vi "LabVIEW-Demo.vi"() -> ()   [LabVIEW 2015]
uses:
  <vilib>/Math Plots/3D Math Plots/3D Scatter/3D Scatter XCtrl/3D Scatter.xctl
  <vilib>/Instr/_visa.llb/VISA Configure Serial Port (Instr).vi
  <vilib>/Math Plots/3D Math Plots/3D Scatter/3D Scatter Datatype/Public/Plot Helper (Vector).vi
  <vilib>/Math Plots/3D Math Plots/3D Scatter/3D Scatter Datatype/3D Scatter Datatype.lvclass
panel:
  in  "milliseconds to wait":u32=50
  out "3D Scatter":refnum<class "3D Plot Datatype.lvclass">[](xcontrol)
  out "zmin":dbl
  out "ymin":dbl
  out "xmin":dbl
  in  "Reset":bool
  out "zmax":dbl
  out "ymax":dbl
  out "xmax":dbl
  out "Temperature Chart":dbl(graph)
  out "Magneticfield Chart":cluster{dbl, dbl, dbl}(graph)
  in  "stop":bool
  in  "VISA resource name":refnum<visa-resource-name>
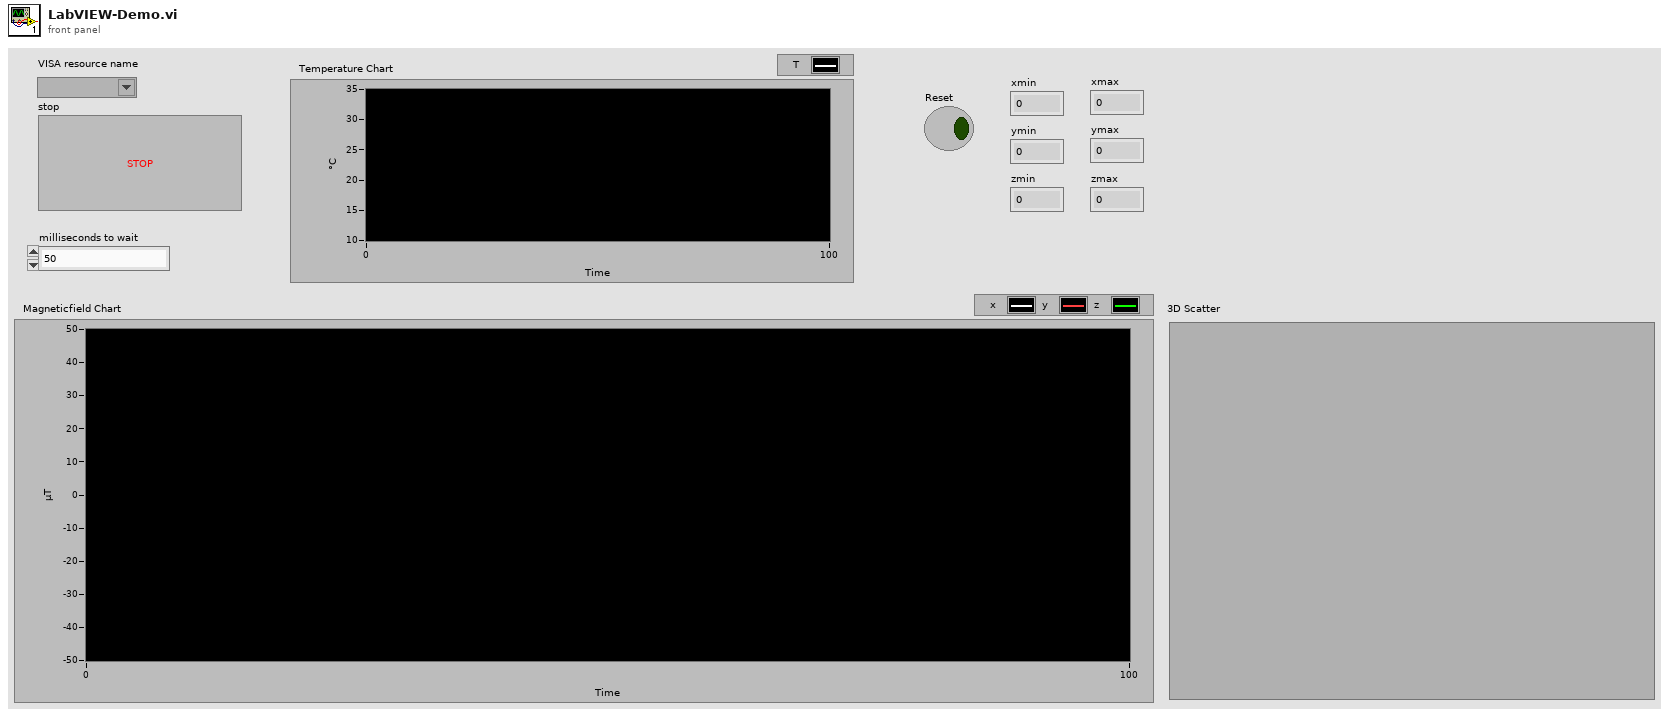
[diagram p1: front panel]
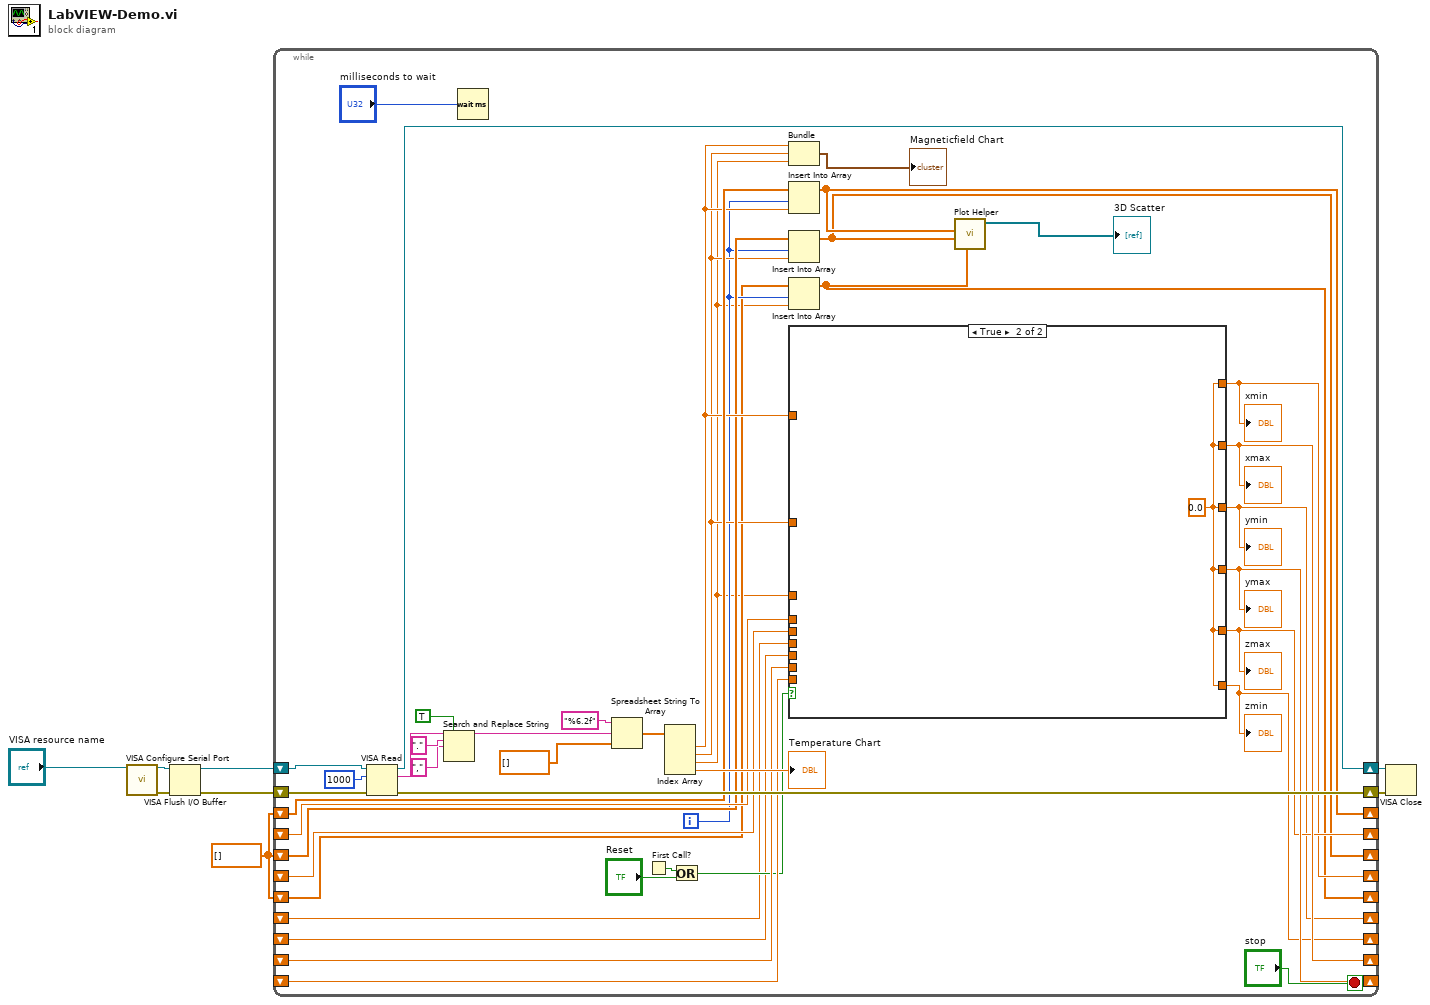
[diagram p0: block diagram]
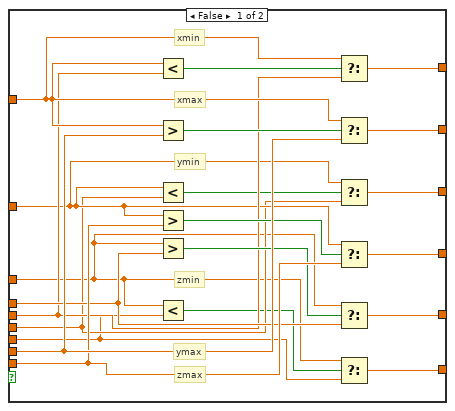
[diagram p2: hidden frame]
diagram:
  w1 = dbl[] [] ("array")
  n1 = call-poly "VISA Configure Serial Port"("VISA resource name"="VISA resource name") -> ("VISA resource name out"=w6:refnum<visa-resource-name>, "error out"=w7:errorcluster)  [unwired: 13 in]
  n2 = VISA Flush I/O Buffer(VISA resource name=w6, error in (no error)=w7) -> (VISA resource name out=w5:refnum<visa-resource-name>, error out=w4:errorcluster)  [unwired: 1 in]
  n3 = while {
    shift-right: [w49] -> w3
    shift-left: w5 -> [w51]
    shift-right: [w48] -> w2
    shift-left: w4 -> [w50]
    shift-right: [w34] -> _
    shift-left: _ -> [w35]
    shift-right: [w31] -> _
    shift-left: _ -> [w33]
    shift-right: [w30] -> _
    shift-left: _ -> [w32]
    shift-right: [w26] -> _
    shift-left: _ -> [w25]
    shift-right: [w24] -> _
    shift-left: _ -> [w23]
    shift-right: [w22] -> _
    shift-left: _ -> [w21]
    shift-right: [w16] -> _
    shift-left: w1 -> [w18]
    shift-right: [w13] -> _
    shift-left: w1 -> [w15]
    shift-right: [w9] -> _
    shift-left: w1 -> [w11]
    i -> [w12]
    stop <- "stop" stop-if-true
    n4 = VISA Read(VISA resource name=w51, byte count=u32 1000, error in (no error)=w50) -> (VISA resource name out=w49:refnum<visa-resource-name>, read buffer=w41:string, error out=w48:errorcluster)  [unwired: 1 out]
    n5 = Search and Replace String(replace all?=TRUE ("replace all? (F)"), input string=w41, search string=".", replace string="," ("replace string (\"\")")) -> (result string=w40:string)  [unwired: 4 in, 3 out]
    n6 = Wait (ms)(milliseconds to wait="milliseconds to wait") -> ()  [unwired: 1 out]
    n7 = Spreadsheet String To Array(format string="%6.2f", spreadsheet string=w40, array type (2D Dbl)=dbl[] []) -> (array=w38:dbl[])  [unwired: 1 in]
    n8 = First Call?() -> (First Call?: T/F=w29:bool)
    n9 = Index Array(array=w38) -> (element #1=w17:dbl, element #2=w14:dbl, element #3=w10:dbl, element #4=→"Temperature Chart":dbl)  [unwired: 4 in]
    n10 = Or(x=w29, y="Reset") -> (x .or. y?=w28:bool)
    n11 = Bundle(w17, w14, w10) -> (→"Magneticfield Chart":cluster{dbl, dbl, dbl})  [unwired: 1 in]
    n12 = Insert Into Array(array=w18, index=w12, new element=w17) -> (w16:dbl[])
    n13 = Insert Into Array(array=w15, index=w12, new element=w14) -> (w13:dbl[])
    n14 = Insert Into Array(array=w11, index=w12, new element=w10) -> (w9:dbl[])
    n15 = case shown="True" w28 {
      tunnel: w17 -> [w62 _]
      tunnel: w35 -> [w71 _]
      tunnel: [w70 w73] -> w34
      tunnel: w14 -> [w58 _]
      tunnel: [w68 w73] -> w31
      tunnel: w33 -> [w67 _]
      tunnel: [w65 w73] -> w30
      tunnel: w10 -> [w52 _]
      tunnel: w32 -> [w64 _]
      tunnel: [w61 w73] -> w26
      tunnel: w25 -> [w60 _]
      tunnel: [w57 w73] -> w24
      tunnel: w23 -> [w56 _]
      tunnel: [w54 w73] -> w22
      tunnel: w21 -> [w53 _]
      frame False {
        # "zmin"
        # "ymin"
        # "xmin"
        # "zmax"
        # "ymax"
        # "xmax"
        n16 = Less?(x=w62, y=w60) -> (x < y?=w63:bool)
        n17 = Greater?(x=w62, y=w71) -> (0:w72:bool)
        n18 = Less?(x=w58, y=w56) -> (x < y?=w59:bool)
        n19 = Greater?(x=w58, y=w67) -> (0:w69:bool)
        n20 = Greater?(x=w52, y=w64) -> (0:w66:bool)
        n21 = Less?(x=w52, y=w53) -> (x < y?=w55:bool)
        n22 = Select(t=w62, s=w63, f=w60) -> (s? t:f=w61:dbl)
        n23 = Select(t=w62, s=w72, f=w71) -> (s? t:f=w70:dbl)
        n24 = Select(t=w58, s=w59, f=w56) -> (s? t:f=w57:dbl)
        n25 = Select(t=w58, s=w69, f=w67) -> (s? t:f=w68:dbl)
        n26 = Select(t=w52, s=w66, f=w64) -> (s? t:f=w65:dbl)
        n27 = Select(t=w52, s=w55, f=w53) -> (s? t:f=w54:dbl)
      }
      frame True {
        w73 = 0.0
      }
    }
    "xmax" <- w34
    "ymax" <- w31
    "zmax" <- w30
    "xmin" <- w26
    "ymin" <- w24
    "zmin" <- w22
    n28 = call-poly <vilib>:"Plot Helper.vi"("z vector"=w9, "y vector"=w13, "x vector"=w16) -> ("3D Plot lvclass Array out"=→"3D Scatter":refnum<class "3D Plot Datatype.lvclass">[])  [unwired: 3 in, 5 out]
  }
  n29 = VISA Close(VISA resource name=w3, error in (no error)=w2) -> ()  [unwired: 1 out]
